vi "InitializationCommunication.vi"(8 "error in":errorcluster, 9 "Cluster of Z settings":T1={"VISA resource name"="COM6", "Channel"=0.0, "Baud Rate (9600)"=9600.0, "Data Bits (8)"=8.0}, 10 "Cluster of Y settings":T1={"VISA resource name"="COM6", "Channel"=0.0, "Baud Rate (9600)"=9600.0, "Data Bits (8)"=8.0}, 11 "Cluster of X settings":T1={"VISA resource name"="COM6", "Channel"=0.0, "Baud Rate (9600)"=9600.0, "Data Bits (8)"=8.0}) -> (0 "error out":errorcluster)   [LabVIEW 2020, in "YP PowerControl.lvlib"]
doc: "_____\nCreated using DQMH Event Scripter 6.0.0.122."
uses:
  YP PowerControl.lvlib
  InitializationCommunication Argument--cluster.ctl
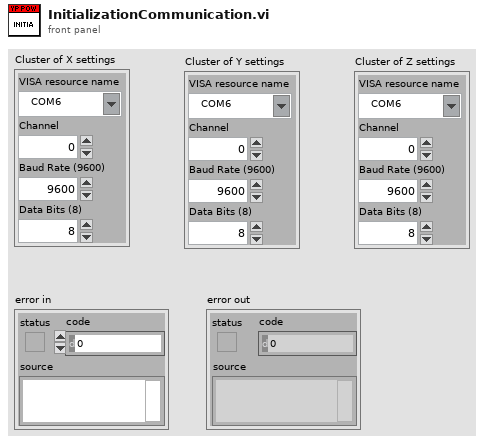
[diagram p1: front panel]
types:
  T1 = cluster{"VISA resource name":refnum<visa-resource-name>, "Channel":dbl, "Baud Rate (9600)":dbl, "Data Bits (8)":dbl}
  T2 = typedef "YP PowerControl.lvlib/InitializationCommunication Argument--cluster.ctl" = cluster{"Cluster of X settings":cluster{"VISA resource name":refnum<visa-resource-name>, "Channel":dbl, "Baud Rate (9600)":dbl, "Data Bits (8)":dbl}, "Cluster of Y settings":cluster{"VISA resource name":refnum<visa-resource-name>, "Channel":dbl, "Baud Rate (9600)":dbl, "Data Bits (8)":dbl}, "Cluster of Z settings":cluster{"VISA resource name":refnum<visa-resource-name>, "Channel":dbl, "Baud Rate (9600)":dbl, "Data Bits (8)":dbl}}
  T3 = typedef "YP PowerControl.lvlib/Request Events--cluster.ctl" = cluster{"Stop Module":refnum<user-event>, "Show Panel":refnum<user-event>, "Hide Panel":refnum<user-event>, "Get Module Execution Status":refnum<user-event>, "Show Diagram":refnum<user-event>, "Currents Set":refnum<user-event>, "InitializationCommunication":refnum<user-event>}
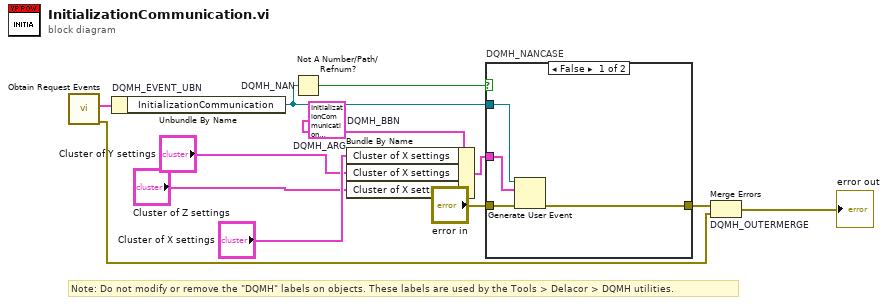
[diagram p0: block diagram]
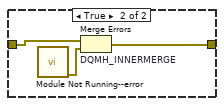
[diagram p2: hidden frame]
diagram:
  w6 = T2 {"Cluster of X settings"={"VISA resource name"="COM6", "Channel"=0.0, "Baud Rate (9600)"=9600.0, "Data Bits (8)"=8.0}, "Cluster of Y settings"={"VISA resource name"="COM6", "Channel"=0.0, "Baud Rate (9600)"=9600.0, "Data Bits (8)"=8.0}, "Cluster of Z settings"={"VISA resource name"="COM6", "Channel"=0.0, "Baud Rate (9600)"=9600.0, "Data Bits (8)"=8.0}}  # DQMH_ARG
  # "Note: Do not modify or remove the \"DQMH\" labels on objects. These labels are used by the Tools > Delacor > DQMH utilities."
  n1 = call "Obtain Request Events.vi"() -> ("error out"=w4:errorcluster, "YP PowerControl Request Events"=w3:T3)  [unwired: 10 in]
  n2 = Unbundle By Name "DQMH_EVENT_UBN"(w3) -> ("InitializationCommunication"=w8:refnum<user-event>)
  n3 = Not A Number/Path/Refnum? "DQMH_NAN"(number/path/refnum=w8) -> (NaN/Path/Refnum?=w9:bool)
  n4 = Bundle By Name "DQMH_BBN"(cluster=w6, "Cluster of X settings"="Cluster of X settings", "Cluster of X settings"="Cluster of Y settings", "Cluster of X settings"="Cluster of Z settings") -> (w10:T2)
  n5 = case "DQMH_NANCASE" shown="False" w9 {
    tunnel: "error in" -> [w16 w19]
    tunnel: [w15 w18] -> w7
    tunnel: w8 -> [w14 _]
    tunnel: w10 -> [w13 _]
    frame False {
      n6 = Generate User Event(user event=w14, event data cluster=w13, error in=w16) -> (error out=w15:errorcluster)  [unwired: 1 in, 1 out]
    }
    frame True {
      n7 = call "Module Not Running--error.vi"() -> ("error out"=w17:errorcluster)  [unwired: 11 in]
      n8 = Merge Errors "DQMH_INNERMERGE"(w19, w17) -> (w18:errorcluster)
    }
  }
  n9 = Merge Errors "DQMH_OUTERMERGE"(w7, w4) -> (→"error out":errorcluster)
